vi "Find Units.vi"(8 "error in":errorcluster, 11 "ParseGDSII in":refnum<class "ParseGDSII.lvclass">) -> (0 "error out":errorcluster, 2 "Scaling Factor":dbl, 3 "ParseGDSII out":refnum<class "ParseGDSII.lvclass">)   [LabVIEW 2019, in "ParseGDSII.lvclass"]
uses:
  ParseGDSII.lvclass
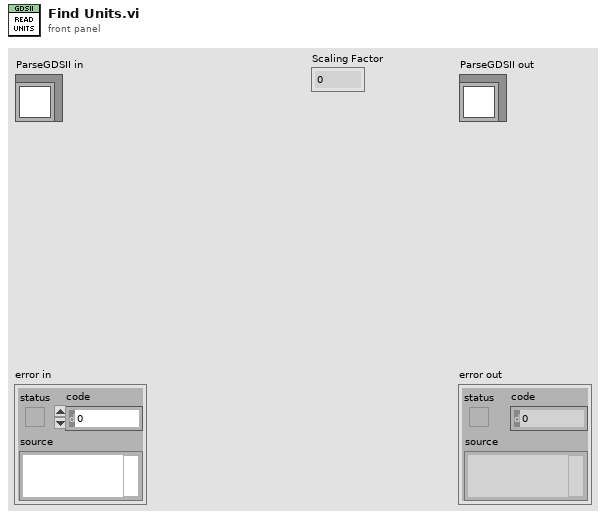
[diagram p1: front panel]
types:
  T1 = cluster{"Record Type":string, "Payload":string, "Parent Index":i32, "First Child Index":i32, "Next Sibling Index":i32}[]
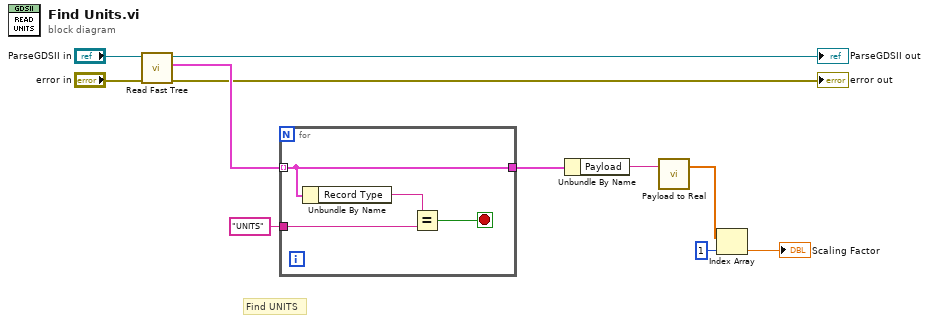
[diagram p0: block diagram]
diagram:
  # "Find UNITS"
  n1 = call "Read Fast Tree.vi"("error in"="error in", "ParseGDSII in"="ParseGDSII in") -> ("error out"=→"error out":errorcluster, "Tree"=w9:T1, "ParseGDSII out"=→"ParseGDSII out":refnum<class "ParseGDSII.lvclass">)  [unwired: 6 in, 1 out]
  n2 = for {
    tunnel: w9 -> [w13] mode=indexing
    tunnel: "UNITS" ("Key") -> [w15]
    tunnel: [w13] -> w7
    stop <- w12 stop-if-true
    n3 = Unbundle By Name(w13) -> ("Record Type"=w14:string)
    n4 = Equal?(x=w14, y=w15) -> (x = y?=w12:bool)
  }
  n5 = Unbundle By Name(w7) -> ("Payload"=w6:string)
  n6 = call "Payload to Real.vi"("Payload"=w6) -> ("Real"=w3:dbl[])  [unwired: 2 in]
  n7 = Index Array(array=w3, index=1) -> (element=→"Scaling Factor":dbl)
